vi "Create Process from File.vi"(8 "error in (no error)":errorcluster, 10 "Process":path, 11 "Process Model in":refnum<class "Process Model.lvclass">) -> (0 "error out":errorcluster, 3 "Process Model out":refnum<class "Process Model.lvclass">)   [LabVIEW 2017, in "Process Model.lvlib" / "Process Model.lvclass"]
uses:
  <vilib>/gpm_packages/@cs/Car wash/Process Model/Process Model/Process Model.lvclass
  <vilib>/gpm_packages/@cs/test-executive/Source/Test Executive/TestExecutive Ref/TestExecutive Ref.lvclass
  <vilib>/gpm_packages/@cs/test-executive/Source/Test Executive/TestExecutive/Test Executive.lvclass
  <vilib>/gpm_packages/@cs/Car wash/gpm_packages/@cs/linked-list/Source/Persistence/XML/XML.lvclass
  C:/Program Files/National Instruments/LabVIEW 2017/vi.lib/gpm_packages/@cs/test-executive/Source/Test Executive/ITestExecutive/ITest Executive.lvclass
  <vilib>/gpm_packages/@cs/persistence/source/IPersist/IPersist.lvclass
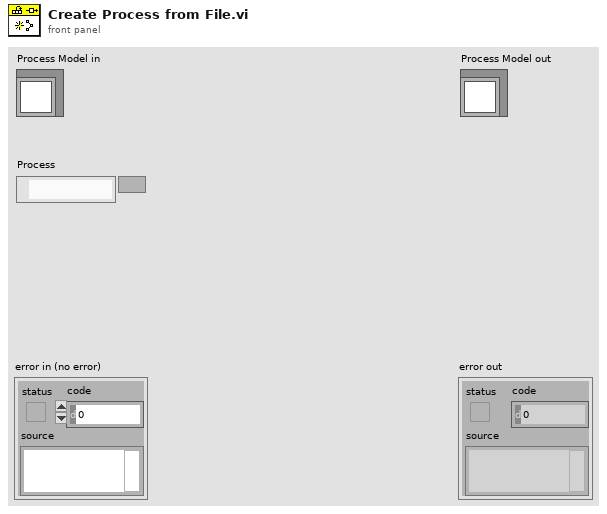
[diagram p1: front panel]
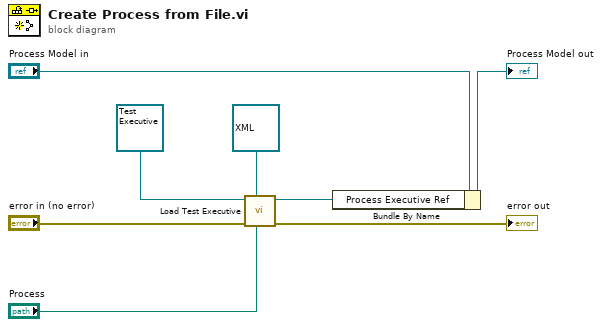
[diagram p0: block diagram]
diagram:
  n1 = call <vilib>:"Load Test Executive.vi"("Folder"="Process", "Persistence in"=refnum<class "XML.lvclass"> refnum ("Linked Lists.lvlib:XML.lvclass"), "error in (no error)"="error in (no error)", "Test Executive"=refnum<class "Test Executive.lvclass"> refnum ("Test Executive.lvlib:Test Executive.lvclass")) -> ("error out"=→"error out":errorcluster, "Test Executive Ref out"=w3:refnum<data-value>)  [unwired: 5 in, 1 out]
  n2 = Bundle By Name(cluster="Process Model in", "Process Executive Ref"=w3) -> (→"Process Model out":refnum<class "Process Model.lvclass">)
